vi "AH_CmdCABLE.vi"(5 "Arg":dbl, 7 "Tries":i32=5, 8 "error in (no error)":errorcluster, 9 "Property":T1(ring), 10 "Data Cluster In":T2 {"GUI Data Cluster"."SBR" format="%08b"}, 11 "Config Cluster In":T4={"General"={"Config.ini"=path "", "Default Logging Path"=path ""}, "Hardware"={"AHC VISA COM"="", "Measure Rate (1/s)"=0, "Global T VAR"="", "Global B VAR"="", "Average"=4, "Bias"=0, "Cable"={"Length"=0.0, "Resistance"=0.0, "Inductance"=0.0, "Capacitance"=0.0}, "Tracking"=0, "Voltage"=0.0}, "Operation"={"Operation Mode"=enum."Logging", "Status"="", "NewLog?"=FALSE}}) -> (0 "error IO":errorcluster, 2 "Data Cluster Out":T2 {"GUI Data Cluster"."SBR" format="%08b"}, 3 "Configuration Cluster Out":T4={"General"={"Config.ini"=path "", "Default Logging Path"=path ""}, "Hardware"={"AHC VISA COM"="", "Measure Rate (1/s)"=0, "Global T VAR"="", "Global B VAR"="", "Average"=4, "Bias"=0, "Cable"={"Length"=0.0, "Resistance"=0.0, "Inductance"=0.0, "Capacitance"=0.0}, "Tracking"=0, "Voltage"=0.0}, "Operation"={"Operation Mode"=enum."Idle-Off", "Status"="", "NewLog?"=FALSE}})   [LabVIEW 2021]
uses:
  Config_Cluster.ctl
  Mode_Enum.ctl
  Data_Cluster.ctl
  Measurement_Cluster.ctl
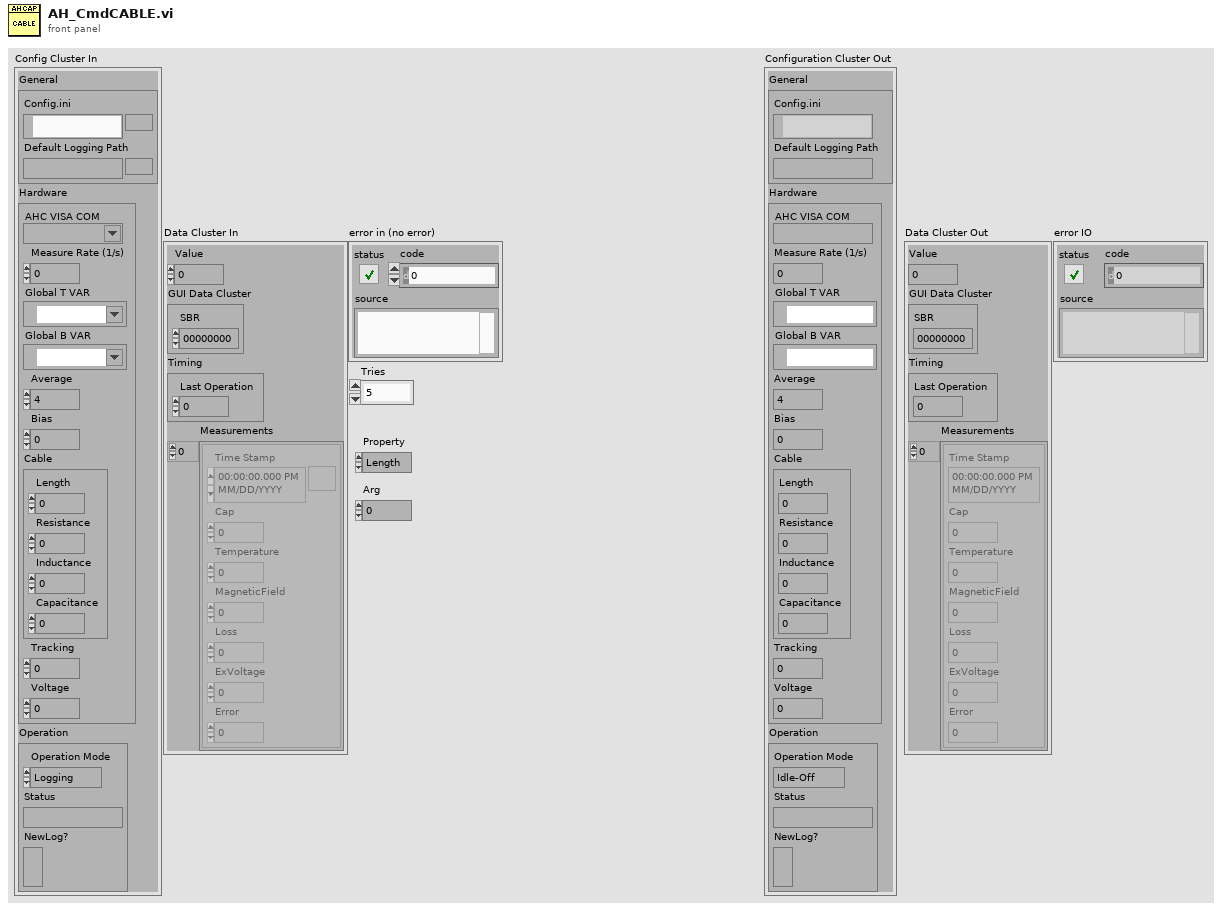
[diagram p1: front panel]
types:
  T1 = enum16{"Length", "Capacitance", "Inductance", "Resistance"}
  T2 = typedef "Data_Cluster.ctl" = cluster{"Value":dbl, "GUI Data Cluster":cluster{"SBR":u16}, "Timing":cluster{"Last Operation":dbl}, "Measurements":T3[]}
  T3 = typedef "Measurement_Cluster.ctl" = cluster{"Time Stamp":timestamp, "Cap":dbl, "Temperature":dbl, "MagneticField":dbl, "Loss":dbl, "ExVoltage":dbl, "Error":dbl}
  T4 = typedef "Config_Cluster.ctl" = cluster{"General":cluster{"Config.ini":path, "Default Logging Path":path}, "Hardware":cluster{"AHC VISA COM":refnum<visa-resource-name>, "Measure Rate (1/s)":i32, "Global T VAR":refnum<k21>, "Global B VAR":refnum<k21>, "Average":u8, "Bias":u8, "Cable":cluster{"Length":dbl, "Resistance":dbl, "Inductance":dbl, "Capacitance":dbl}, "Tracking":u8, "Voltage":dbl}, "Operation":cluster{"Operation Mode":T5, "Status":string, "NewLog?":bool}}
  T5 = typedef "Mode_Enum.ctl" = enum16{"Logging", "Idle-Off", "Idle"}
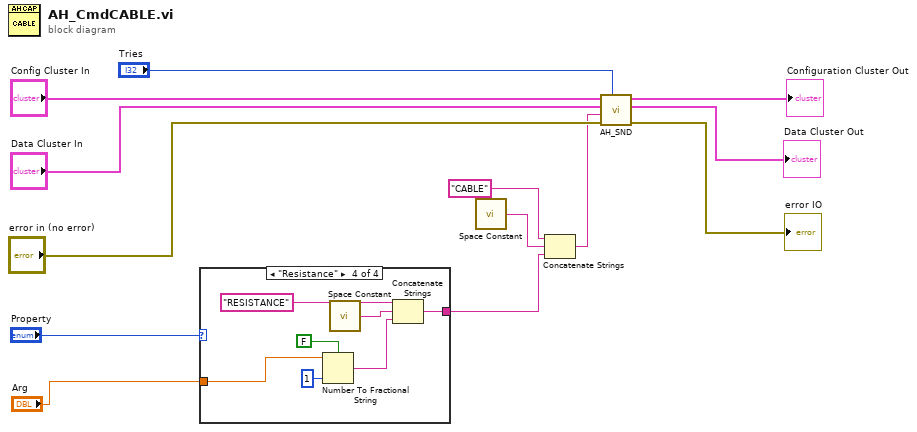
[diagram p0: block diagram]
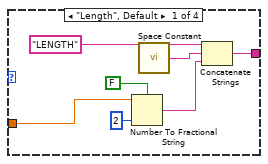
[diagram p2: hidden frame]
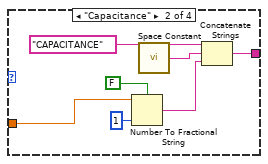
[diagram p3: hidden frame]
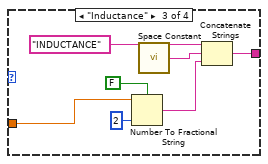
[diagram p4: hidden frame]
diagram:
  n1 = case shown="\"Resistance\"" "Property" {
    tunnel: "Arg" -> [w20 w27 w34 w41]
    tunnel: [w14 w21 w28 w35] -> w1
    frame "Length", Default {
      n2 = Number To Fractional String(use system decimal point (T)=FALSE, number=w20, precision (6)=i16 2) -> (F-format string=w15:string)  [unwired: 1 in]
      n3 = call <vilib>:"Space Constant.vi"() -> ("String"=w16:string)
      n4 = Concatenate Strings("LENGTH", w16, w15) -> (w14:string)
    }
    frame "Capacitance" {
      n5 = Number To Fractional String(use system decimal point (T)=FALSE, number=w27, precision (6)=i16 1) -> (F-format string=w22:string)  [unwired: 1 in]
      n6 = call <vilib>:"Space Constant.vi"() -> ("String"=w23:string)
      n7 = Concatenate Strings("CAPACITANCE", w23, w22) -> (w21:string)
    }
    frame "Inductance" {
      n8 = Number To Fractional String(use system decimal point (T)=FALSE, number=w34, precision (6)=i16 2) -> (F-format string=w29:string)  [unwired: 1 in]
      n9 = call <vilib>:"Space Constant.vi"() -> ("String"=w30:string)
      n10 = Concatenate Strings("INDUCTANCE", w30, w29) -> (w28:string)
    }
    frame "Resistance" {
      n11 = Number To Fractional String(use system decimal point (T)=FALSE, number=w41, precision (6)=i16 1) -> (F-format string=w36:string)  [unwired: 1 in]
      n12 = call <vilib>:"Space Constant.vi"() -> ("String"=w37:string)
      n13 = Concatenate Strings("RESISTANCE", w37, w36) -> (w35:string)
    }
  }
  n14 = call <vilib>:"Space Constant.vi"() -> ("String"=w9:string)
  n15 = Concatenate Strings("CABLE", w9, w1) -> (w7:string)
  n16 = call "AH_SND.vi"("Tries"="Tries", "error in (no error)"="error in (no error)", "CMD"=w7, "Data Cluster In"="Data Cluster In", "Config Cluster In"="Config Cluster In") -> ("error IO"=→"error IO":errorcluster, "Data Cluster Out"=→"Data Cluster Out":T2, "Configuration Cluster Out"=→"Configuration Cluster Out":T4)  [unwired: 4 in]
